vi "Simple Add.vi"() -> ()   [LabVIEW 2018]
panel:
  out "Numeric Indicator":dbl
  in  "Numeric Control 2":dbl
  in  "Numeric Control":dbl
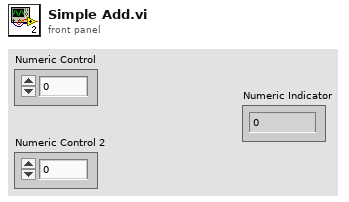
[diagram p1: front panel]
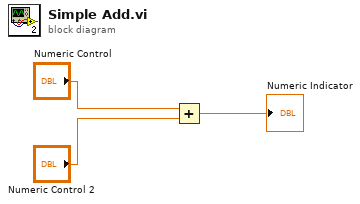
[diagram p0: block diagram]
diagram:
  n1 = Add(x="Numeric Control", y="Numeric Control 2") -> (x+y=→"Numeric Indicator":dbl)
